vi "Move piezo slow.vi"(7 "error in (no error)":errorcluster, 8 "MOVE TO [MICRON]":dbl=1.0 format="%0.2f", 9 "notifier out":refnum<notifier>, 10 "Hardware Configuration":T1) -> (0 "error out":errorcluster, 3 "Hardware Configuration 2":T1)   [LabVIEW 2013]
uses:
  Hardware Configuration Piezo.ctl
  Piezo/Piezo display.ctl
  <vilib>/Analysis/1siggen.llb/Ramp Pattern by Samples.vi
  <vilib>/DAQmx/create/channels.llb/DAQmx Create Channel (AO-Voltage-Basic).vi
  <vilib>/DAQmx/write.llb/DAQmx Write (Analog DBL 1Chan 1Samp).vi
  <vilib>/Analysis/NI_AALBase.lvlib
  Piezo/Piezo.lvlib
panel:
  out "PiezoPosition":sgl
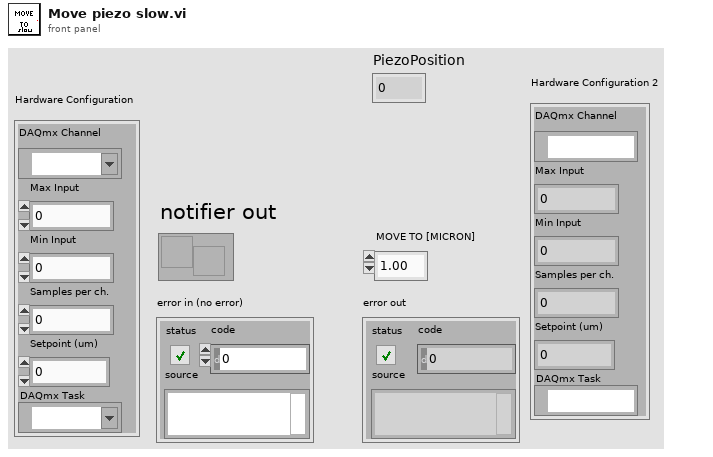
[diagram p1: front panel]
types:
  T1 = typedef "Piezo.lvlib/Hardware Configuration Piezo.ctl" = cluster{"DAQmx Channel":tag, "Max Input":dbl, "Min Input":dbl, "Samples per ch.":dbl, "Setpoint (um)":dbl, "DAQmx Task":refnum<k21>}
  T2 = cluster{"physical channels":tag, "MAX   VOLTAGE":dbl, "MIN   VOLTAGE":dbl}
  T3 = typedef "Piezo.lvlib/Piezo display.ctl" = cluster{"PiezoPosition":sgl, "Counter Time":i32}
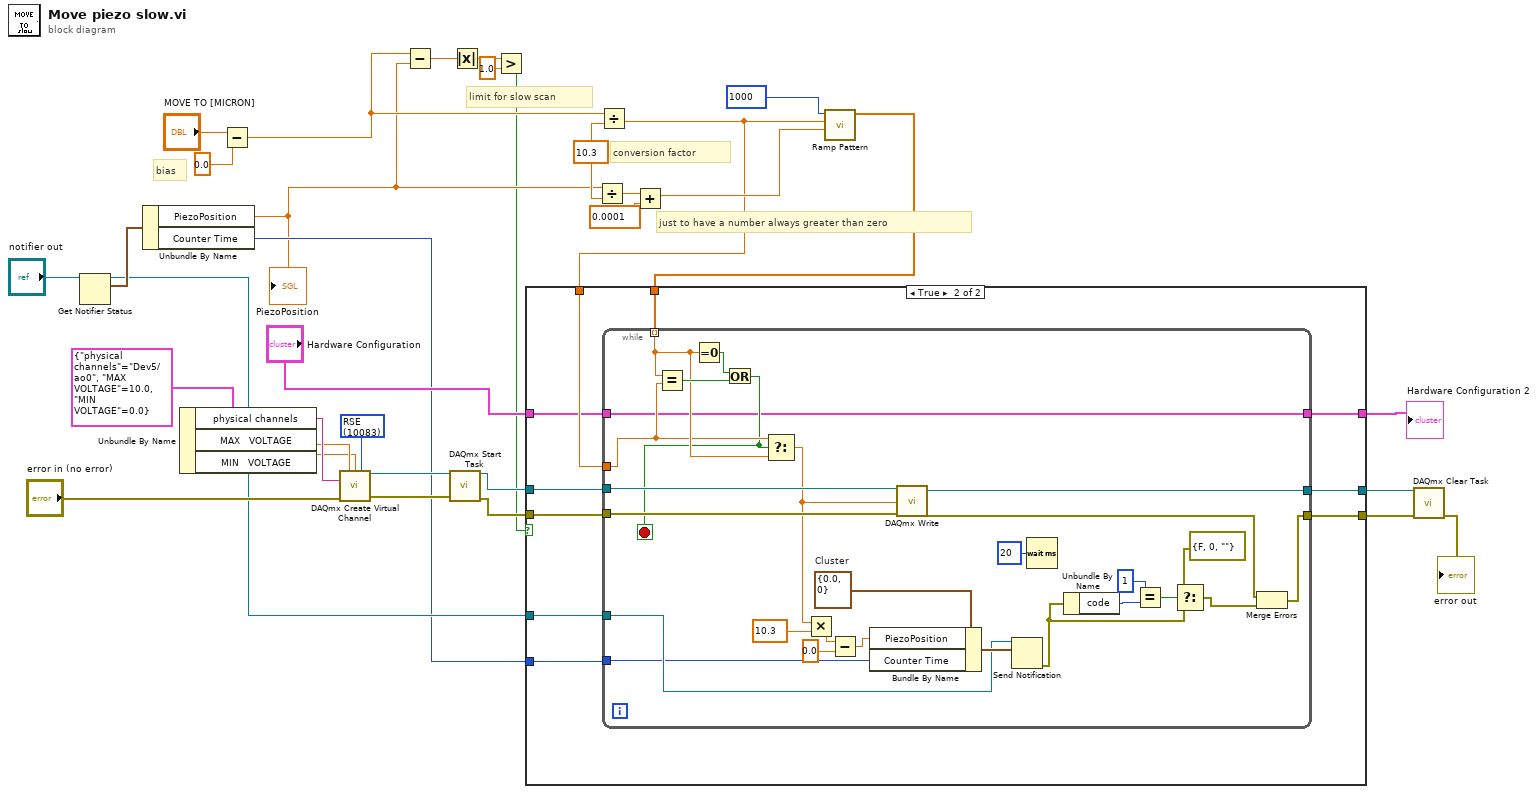
[diagram p0: block diagram]
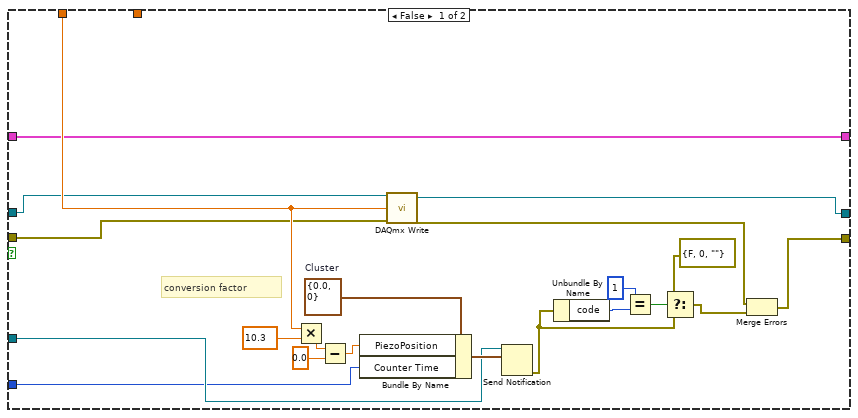
[diagram p2: hidden frame]
diagram:
  w26 = 10083 items=["Default"=-1, "RSE"=10083, "Differential"=10106, "Pseudodifferential"=12529] ("output terminal configuration")
  w31 = 10.3
  # "limit for slow scan"
  # "just to have a number always greater than zero"
  # "bias"
  # "conversion factor"
  n1 = Get Notifier Status(notifier="notifier out") -> (notifier out=w11:refnum<notifier>, current notification=w27:T3)  [unwired: 1 in, 3 out]
  n2 = Unbundle By Name(w27) -> ("PiezoPosition"=w2:sgl, "Counter Time"=w10:i32)
  "PiezoPosition" <- w2
  n3 = Unbundle By Name(T2 {"physical channels"="Dev5/ao0", "MAX   VOLTAGE"=10.0, "MIN   VOLTAGE"=0.0} ("Cluster")) -> ("physical channels"=w22:tag, "MAX   VOLTAGE"=w21:dbl, "MIN   VOLTAGE"=w20:dbl)
  n4 = Subtract(x="MOVE TO [MICRON]", y=0.0) -> (x-y=w3:dbl)
  n5 = call-poly <vilib>:"DAQmx Create Virtual Channel.vi"("maximum value"=w21, "minimum value"=w20, "output terminal configuration"=w26, "physical channels"=w22, "error in"="error in (no error)") -> ("task out"=w25:refnum<k21>, "error out"=w24:errorcluster)  [unwired: 9 in]
  n6 = Subtract(x=w3, y=w2) -> (x-y=w6:dbl)
  n7 = call <vilib>:"DAQmx Start Task.vi"("task/channels in"=w25, "error in"=w24) -> ("task out"=w16:refnum<k21>, "error out"=w15:errorcluster)  [unwired: 12 in]
  n8 = Absolute Value(x=w6) -> (abs(x)=w5:dbl)
  n9 = Greater?(x=w5, y=1.0) -> (0:w1:bool)
  n10 = Divide(x=w2, y=w31) -> (x/y=w32:dbl)
  n11 = Divide(x=w3, y=w31) -> (x/y=w29:dbl)
  n12 = Add(x=w32, y=0.0001) -> (x+y=w33:dbl)
  n13 = call-poly <vilib>:"Ramp Pattern.vi"("start"=w33, "end"=w29, "samples"=1000) -> ("Ramp Pattern"=w30:dbl[])  [unwired: 7 in, 1 out]
  n14 = case shown="True" w1 {
    tunnel: w30 -> [_ w65]
    tunnel: w29 -> [w42 w64]
    tunnel: [w39 w63] -> w18
    tunnel: [w38 w62] -> w17
    tunnel: w16 -> [w41 w61]
    tunnel: w15 -> [w40 w60]
    tunnel: "Hardware Configuration" -> [w35 w59]
    tunnel: [w35 w58] -> w12
    tunnel: w11 -> [w37 w57]
    tunnel: w10 -> [w36 w56]
    frame False {
      w54 = T3 {"PiezoPosition"=0.0, "Counter Time"=0}  # Cluster
      # "conversion factor"
      n15 = Multiply(x=w42, y=10.3) -> (x*y=w44:dbl)
      n16 = Subtract(x=w44, y=0.0) -> (x-y=w45:dbl)
      n17 = Bundle By Name(cluster=w54, "PiezoPosition"=w45, "Counter Time"=w36) -> (w55:T3)
      n18 = call-poly <vilib>:"DAQmx Write.vi"("task/channels in"=w41, "data"=w42, "error in"=w40) -> ("task out"=w39:refnum<k21>, "error out"=w49:errorcluster)  [unwired: 10 in, 1 out]
      n19 = Send Notification(notification=w55, notifier=w37) -> (error out=w48:errorcluster)  [unwired: 1 in, 1 out]
      n20 = Unbundle By Name(w48) -> ("code"=w53:i32)
      n21 = Equal?(x=1, y=w53) -> (x = y?=w51:bool)
      n22 = Select(t=errorcluster {"status"=FALSE, "code"=0, "source"=""} ("error constant"), s=w51, f=w48) -> (s? t:f=w47:errorcluster)
      n23 = Merge Errors(w49, w47) -> (w38:errorcluster)
    }
    frame True {
      n24 = while {
        tunnel: w61 -> [w92]
        tunnel: w60 -> [w91]
        tunnel: [w90] -> w63
        tunnel: [w71] -> w62
        tunnel: w65 -> [w87] mode=indexing
        tunnel: w64 -> [w86]
        tunnel: w59 -> [w83]
        tunnel: [w83] -> w58
        tunnel: w57 -> [w81]
        tunnel: w56 -> [w79]
        stop <- w85 stop-if-true
        w80 = T3 {"PiezoPosition"=0.0, "Counter Time"=0}  # Cluster
        n25 = Equal?(x=w87, y=w86) -> (x = y?=w88:bool)
        n26 = Equal To 0?(x=w87) -> (x = 0?=w89:bool)
        n27 = Or(x=w89, y=w88) -> (x .or. y?=w85:bool)
        n28 = Select(t=w86, s=w85, f=w87) -> (s? t:f=w69:dbl)
        n29 = Multiply(x=w69, y=10.3) -> (x*y=w67:dbl)
        n30 = Subtract(x=w67, y=0.0) -> (x-y=w68:dbl)
        n31 = Bundle By Name(cluster=w80, "PiezoPosition"=w68, "Counter Time"=w79) -> (w82:T3)
        n32 = call-poly <vilib>:"DAQmx Write.vi"("task/channels in"=w92, "data"=w69, "error in"=w91) -> ("task out"=w90:refnum<k21>, "error out"=w74:errorcluster)  [unwired: 10 in, 1 out]
        n33 = Send Notification(notification=w82, notifier=w81) -> (error out=w73:errorcluster)  [unwired: 1 in, 1 out]
        n34 = Wait (ms)(milliseconds to wait=u32 20) -> ()  [unwired: 1 out]
        n35 = Unbundle By Name(w73) -> ("code"=w78:i32)
        n36 = Equal?(x=1, y=w78) -> (x = y?=w76:bool)
        n37 = Select(t=errorcluster {"status"=FALSE, "code"=0, "source"=""} ("error constant"), s=w76, f=w73) -> (s? t:f=w72:errorcluster)
        n38 = Merge Errors(w74, w72) -> (w71:errorcluster)
      }
    }
  }
  "Hardware Configuration 2" <- w12
  n39 = call <vilib>:"DAQmx Clear Task.vi"("task in"=w18, "error in"=w17) -> ("error out"=→"error out":errorcluster)  [unwired: 13 in]
